vi "Agilent_Read Actual Record Length.vi"(8 "error in (no error)":errorcluster, 11 "VISA resource name":refnum<visa-resource-name>) -> (0 "error out":errorcluster, 2 "Actual Record Length":i32, 3 "VISA resource name out":refnum<visa-resource-name>)   [LabVIEW 2009]
doc: "This VI returns the actual number of points the oscilloscope acquires for each channel. After you configure the oscilloscope for an acquisition, call this VI to determine the size of the waveforms that the oscilloscope acquires. The value is equal to or greater than the minimum number of points you specify in the ag6000a Configure Acquisition Record.vi. \n\nNotes:\n(1) The oscilloscope may use different size records depending on the acquisition type. You specify the acquisition type with the ag6000a Configure Acquisition Type.vi."
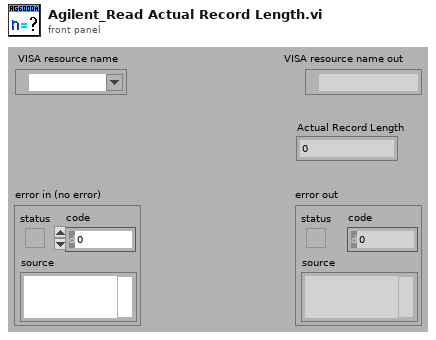
[diagram p1: front panel]
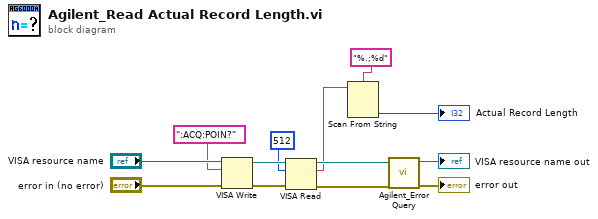
[diagram p0: block diagram]
diagram:
  n1 = VISA Write(VISA resource name="VISA resource name", write buffer=":ACQ:POIN?", error in (no error)="error in (no error)") -> (VISA resource name out=w5:refnum<visa-resource-name>, error out=w8:errorcluster)  [unwired: 1 out]
  n2 = VISA Read(VISA resource name=w5, byte count=u32 512, error in (no error)=w8) -> (VISA resource name out=w6:refnum<visa-resource-name>, read buffer=w3:string, error out=w7:errorcluster)  [unwired: 1 out]
  n3 = Scan From String(format string="%.;%d", input string=w3) -> (output 1=→"Actual Record Length":i32)  [unwired: 3 in, 3 out]
  n4 = call "Agilent_Error Query.vi"("error in (no error)"=w7, "VISA resource name"=w6) -> ("error out"=→"error out":errorcluster, "VISA resource name out"=→"VISA resource name out":refnum<visa-resource-name>)  [unwired: 6 in, 2 out]
